vi "Dictionary to Indicator.vi"(0 "Results.Results (Dictionary)":cluster{"key":string, "value":dbl}[](array[cluster]), 5 "AI Channel":i32=1 max=7 step=1, 11 "error in (no error)":errorcluster) -> (4 "X":dbl, 6 "Y":dbl, 8 "R":dbl, 10 "Theta":dbl, 15 "error out":errorcluster)   [LabVIEW 2016, in "Instrument.Lockin.lvclass"]
uses:
  Instrument.Lockin.lvclass
  Typedefs/Results Type--Enum.ctl
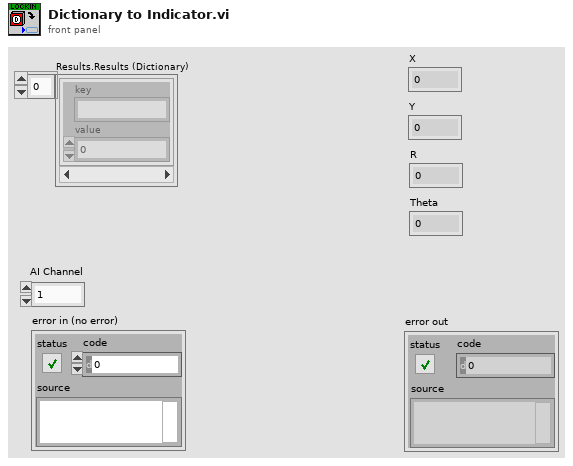
[diagram p1: front panel]
types:
  T1 = typedef "Instrument.Lockin.lvclass/Results Type--Enum.ctl" = enum16{"X", "Y", "R", "Theta", "Mean"}
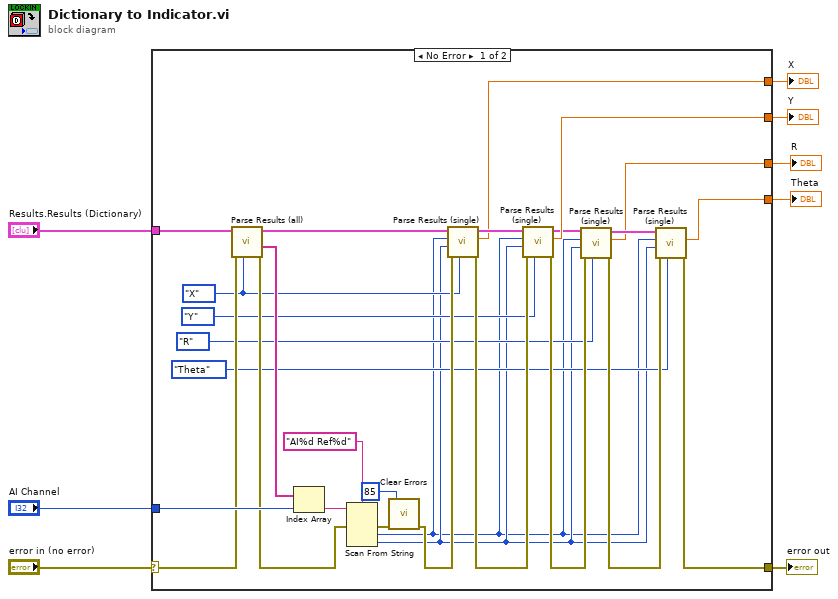
[diagram p0: block diagram]
diagram:
  n1 = case shown="No Error" "error in (no error)" {
    selector: "error in (no error)" -> [w22 w37]
    tunnel: "Results.Results (Dictionary)" -> [w36 _]
    tunnel: "AI Channel" -> [w30 _]
    tunnel: [w32 _] -> w6
    tunnel: [w33 _] -> w5
    tunnel: [w17 w37] -> w3
    tunnel: [w10 _] -> w1
    tunnel: [w9 _] -> w2
    frame No Error {
      w21 = Results_Type--Enum."X" ("Type")
      n2 = call "Parse Results (all).vi"("Type"=w21, "error in (no error)"=w22, "Results (Dictionary)"=w36) -> ("error out"=w28:errorcluster, "Names"=w27:string[], "Results (Dictionary)"=w35:cluster{"key":string, "value":dbl}[])  [unwired: 5 in, 1 out]
      n3 = Index Array(array=w27, index=w30) -> (element=w29:string)
      n4 = Scan From String(format string="AI%d Ref%d", input string=w29, error in=w28) -> (error out=w25:errorcluster, output 1=w11:i32, output 2=w12:i32)  [unwired: 3 in, 2 out]
      n5 = call <vilib>:"Clear Errors.vi"("error in (no error)"=w25, "specific error code to clear (0: all)"=85) -> ("error out"=w24:errorcluster)  [unwired: 4 in, 1 out]
      n6 = call "Parse Results (single).vi"("Type"=w21, "error in (no error)"=w24, "Reference Channel"=w12, "AI Channel"=w11, "Results (Dictionary)"=w35) -> ("error out"=w31:errorcluster, "Data"=w32:dbl, "Results (Dictionary)"=w34:cluster{"key":string, "value":dbl}[])  [unwired: 3 in, 1 out]
      n7 = call "Parse Results (single).vi"("Type"=Results_Type--Enum."Y", "error in (no error)"=w31, "Reference Channel"=w12, "AI Channel"=w11, "Results (Dictionary)"=w34) -> ("error out"=w19:errorcluster, "Data"=w33:dbl, "Results (Dictionary)"=w14:cluster{"key":string, "value":dbl}[])  [unwired: 3 in, 1 out]
      n8 = call "Parse Results (single).vi"("Type"=Results_Type--Enum."R", "error in (no error)"=w19, "Reference Channel"=w12, "AI Channel"=w11, "Results (Dictionary)"=w14) -> ("error out"=w18:errorcluster, "Data"=w10:dbl, "Results (Dictionary)"=w20:cluster{"key":string, "value":dbl}[])  [unwired: 3 in, 1 out]
      n9 = call "Parse Results (single).vi"("Type"=Results_Type--Enum."Theta", "error in (no error)"=w18, "Reference Channel"=w12, "AI Channel"=w11, "Results (Dictionary)"=w20) -> ("error out"=w17:errorcluster, "Data"=w9:dbl)  [unwired: 3 in, 2 out]
    }
    frame Error {
    }
  }
  "X" <- w6
  "Y" <- w5
  "error out" <- w3
  "R" <- w1
  "Theta" <- w2
